vi "pattern_match_subvi.vi"(0 "Match Image In":T1, 1 "Settings":T5={"Curve Parameters"={"Extraction Mode"=0, "Edge Threshold"=30, "Edge Filter Size"=1, "Min Length"=25, "Row Search Step Size"=5, "Col Search Step Size"=2, "Max Endpoint Gap"=10, "Closed"=FALSE, "Subpixel"=FALSE}, "Match Mode"={"Rotation"=TRUE, "Scale"=FALSE, "Occlusion"=FALSE, "Reserved"=FALSE, "Reserved"=FALSE, "Reserved"=FALSE}, "Range Settings"=[], "Number of Matches Requested"=1, "Minimum Match Score"=800.0, "Subpixel Accuracy"=FALSE, "Advanced Geometric Match Options 2"=[]} {"Advanced Geometric Match Options 2"."Item Value" format="%.2f"; "Advanced Geometric Match Options 2"."Setup Data Item" items=["Curve Extraction Mode", "Curve Edge Threshold", "Curve Edge Filter Size", "Min Curve Length", "Curve Row Search Step Size", "Curve Col Search Step Size", "Curve Max Endpoint Gap", "Extract Closed Curves", "Enable Subpixel Curve Extraction", "Enable Correlation Score", "Enable Subpixel Accuracy", "Subpixel Iterations", "Subpixel Tolerance", "Initial Match List Length", "Enable Target Template Curve Score", "Min Match Separation Distance", "Min Match Separation Angle", "Min Match Separation Scale", "Max Match Overlap", "Enable Coarse Result", "Enable Calibration Support", "Enable Contrast Reversal", "Search Strategy", "Refinement Match Factor", "Subpixel Match Factor"]; "Minimum Match Score" min=0 max=1000 format="%.2f"; "Number of Matches Requested" min=1; "Range Settings"."Max" format="%.2f"; "Range Settings"."Min" format="%.2f"; "Range Settings"."Match Constraints" items=["Rotation Angle (degrees)", "Scale Factor (%)", "Occlusion (%)"]; "Curve Parameters"."Extraction Mode" items=["Normal", "Uniform Regions"]; "Curve Parameters"."Edge Filter Size" items=["Fine", "Normal", "Contour Tracing"]; "Curve Parameters"."Max Endpoint Gap" min=0; "Curve Parameters"."Col Search Step Size" min=1 max=255 step=1; "Curve Parameters"."Row Search Step Size" min=1 max=255 step=1; "Curve Parameters"."Min Length" min=0; "Curve Parameters"."Edge Threshold" min=1 max=350 step=1}, 5 "Template Image In":T1, 7 "select (false=mod))":bool, 9 "ROI Descriptor":T6 {"Contours"."Type" items=["No Selection", "Point", "Line", "Rectangle", "Oval", "Polygon", "Freehand Region", "Annulus", "Unused2", "Unused3", "Broken Line", "Freehand Line", "Rotated Rectangle"]}, 11 "error in (no error)":errorcluster, 12 "Path In":path) -> (4 "Refnum out":T1, 6 "Number of Matches":i32, 10 "Matches":T2[](array[typedef]) {"Correlation Score" format="%.2f"; "Target Template Curve Score" format="%.2f"; "Template Target Curve Score" format="%.2f"; "Bounding Box"."y" format="%.2f"; "Bounding Box"."x" format="%.2f"; "Position"."y" format="%.2f"; "Position"."x" format="%.2f"; "Score" format="%.2f"; "Scale" format="%.2f"; "Angle" format="%.2f"; "Occlusion %" format="%.2f"}, 15 "error out":errorcluster)   [LabVIEW 2015]
uses:
  <vilib>/vision/Image Controls.llb/IMAQ Image.ctl
  <vilib>/vision/Pattern Matching.llb/IMAQ Curve Parameters.ctl
  <vilib>/vision/Pattern Matching.llb/IMAQ Match Range Setting.ctl
  <vilib>/vision/Pattern Matching.llb/IMAQ GM Match Report.ctl
  <vilib>/vision/NI_Vision_Development_Module.lvlib
panel:
  # "Range"
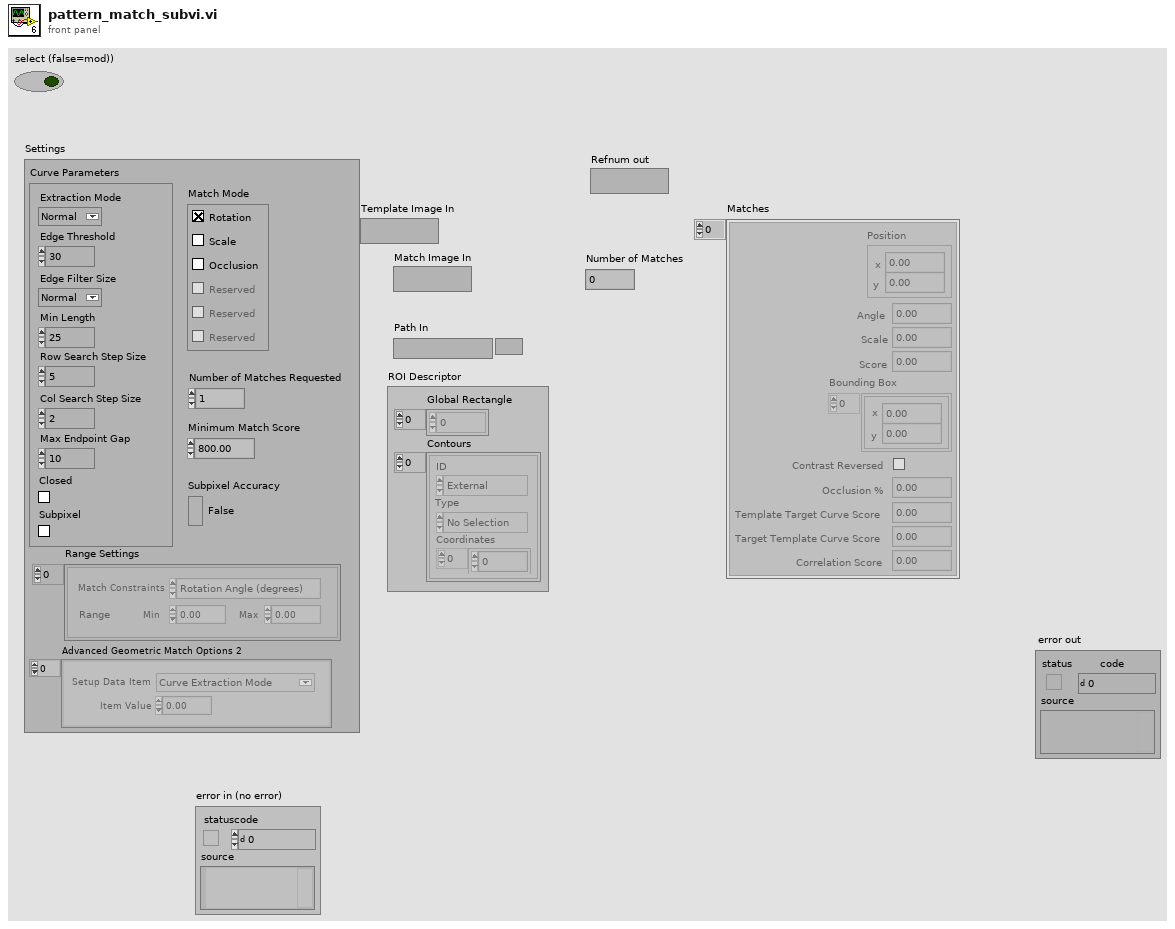
[diagram p1: front panel]
types:
  T1 = typedef "IMAQ Image.ctl" = refnum<image>
  T2 = typedef "IMAQ GM Match Report.ctl" = cluster{"Position":cluster{"x":sgl, "y":sgl}, "Angle":sgl, "Scale":sgl, "Score":sgl, "Bounding Box":cluster{"x":sgl, "y":sgl}[], "Contrast Reversed":bool, "Occlusion %":sgl, "Template Target Curve Score":sgl, "Target Template Curve Score":sgl, "Correlation Score":sgl}
  T3 = typedef "IMAQ Curve Parameters.ctl" = cluster{"Extraction Mode":u32, "Edge Threshold":i32, "Edge Filter Size":u32, "Min Length":i32, "Row Search Step Size":i32, "Col Search Step Size":i32, "Max Endpoint Gap":i32, "Closed":bool, "Subpixel":bool}
  T4 = typedef "IMAQ Match Range Setting.ctl" = cluster{"Match Constraints":u32, "Min":dbl, "Max":dbl}
  T5 = cluster{"Curve Parameters":T3, "Match Mode":cluster{"Rotation":bool, "Scale":bool, "Occlusion":bool, "Reserved":bool, "Reserved":bool, "Reserved":bool}, "Range Settings":T4[], "Number of Matches Requested":i32, "Minimum Match Score":sgl, "Subpixel Accuracy":bool, "Advanced Geometric Match Options 2":cluster{"Setup Data Item":u16, "Item Value":dbl}[]}
  T6 = cluster{"Global Rectangle":i32[], "Contours":cluster{"ID":enum32{"External", "Internal"}, "Type":u32, "Coordinates":i32[]}[]}
  T7 = cluster{"Rotation":bool, "Scale":bool, "Occlusion":bool, "Reserved":bool, "Reserved":bool, "Reserved":bool}
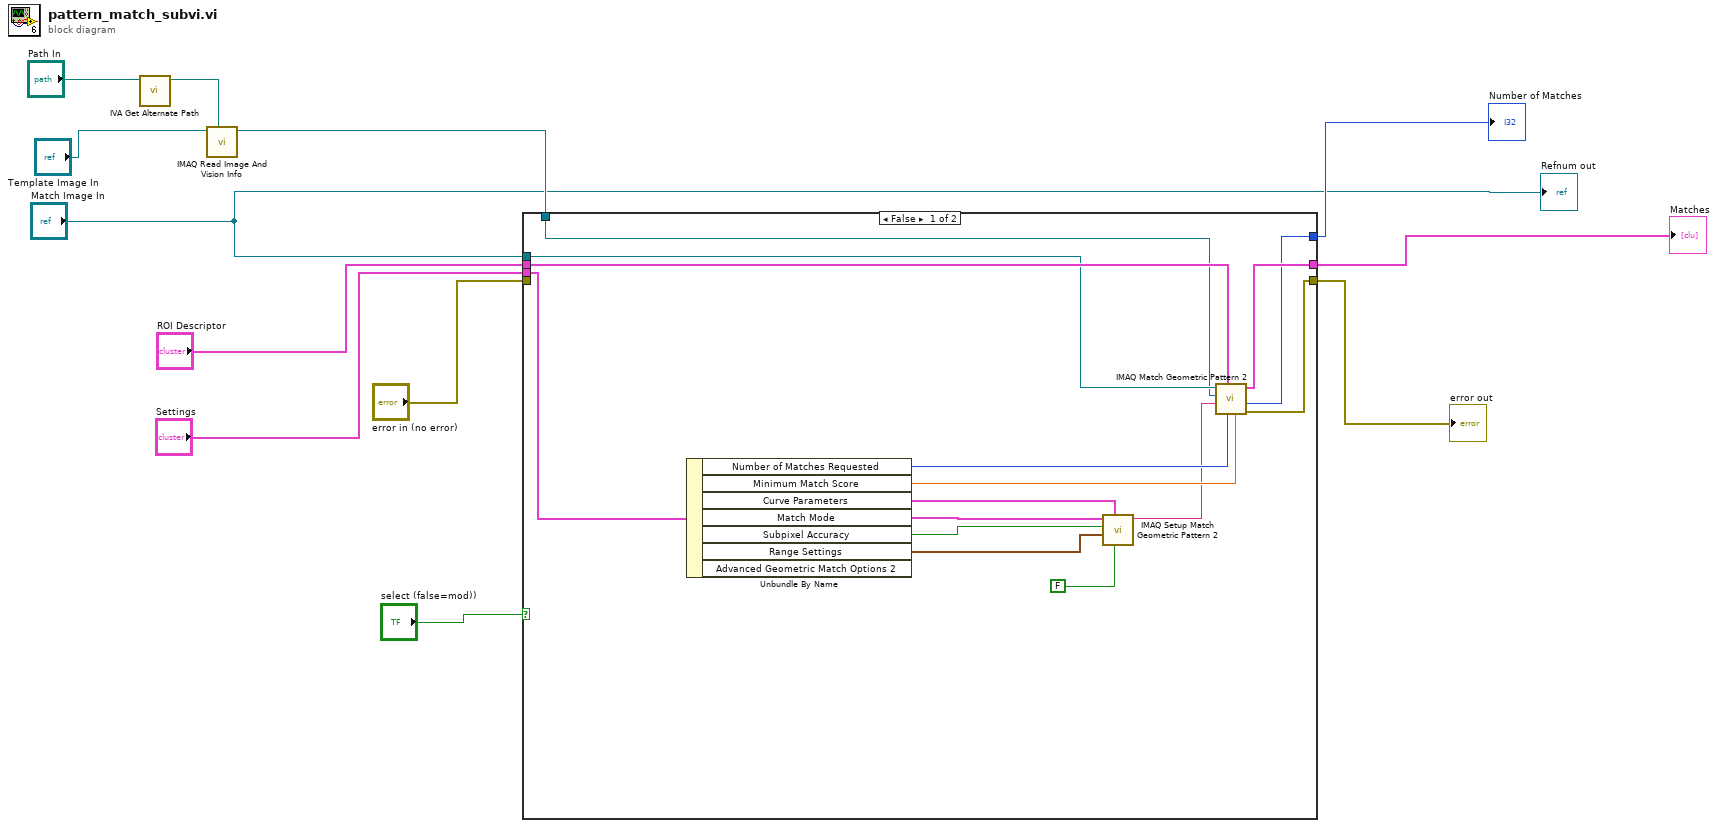
[diagram p0: block diagram]
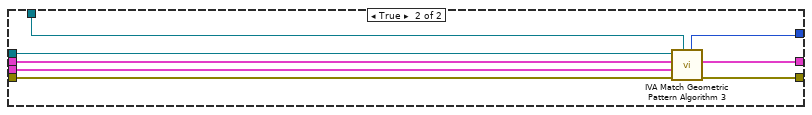
[diagram p2: hidden frame]
diagram:
  n1 = call <vilib>:"IVA Get Alternate Path.vi"("Path In"="Path In") -> ("Path Out"=w5:path)  [unwired: 10 out]
  n2 = call "IMAQ Read Image And Vision Info"("File Path"=w5, "Image"="Template Image In") -> ("Image Out"=w6:T1)  [unwired: 2 in, 7 out]
  n3 = case shown="False" "select (false=mod))" {
    tunnel: "error in (no error)" -> [_ w35]
    tunnel: [w14 w34] -> w10
    tunnel: "Settings" -> [w20 w33]
    tunnel: "ROI Descriptor" -> [w17 w32]
    tunnel: [w19 w31] -> w7
    tunnel: w6 -> [w15 w30]
    tunnel: "Match Image In" -> [w16 w29]
    tunnel: [w18 w28] -> w2
    frame False {
      n4 = Unbundle By Name(w20) -> ("Number of Matches Requested"=w22:i32, "Minimum Match Score"=w21:sgl, "Curve Parameters"=w23:T3, "Match Mode"=w24:T7, "Subpixel Accuracy"=w25:bool, "Range Settings"=w26:T4[])  [unwired: 1 out]
      n5 = call "IMAQ Setup Match Geometric Pattern 2"("Use Learn Curve Parameters"=FALSE, "Curve Parameters"=w23, "Range Settings"=w26, "Subpixel Accuracy"=w25, "Match Mode"=w24) -> ("Match Geometric Pattern 2 Setup Data"=w13:string)  [unwired: 1 in, 5 out]
      n6 = call "IMAQ Match Geometric Pattern 2"("Minimum Match Score"=w21, "Number of Matches Requested"=w22, "ROI Descriptor"=w17, "Match Geometric Pattern 2 Setup Data"=w13, "Template Image"=w15, "Image"=w16) -> ("error out"=w18:errorcluster, "Number of Matches"=w14:i32, "Matches (pixel)"=w19:T2[])  [unwired: 1 in, 2 out]
    }
    frame True {
      n7 = call <vilib>:"IVA Match Geometric Pattern Algorithm 3.vi"("Template"=w30, "error in (no error)"=w35, "Settings"=w33, "ROI Descriptor"=w32, "Image"=w29) -> ("error out"=w28:errorcluster, "Matches"=w31:T2[], "Number of Matches"=w34:i32)  [unwired: 4 out]
    }
  }
  "Number of Matches" <- w10
  "error out" <- w2
  "Matches" <- w7
  "Refnum out" <- "Match Image In"
